vi "PID Online Autotuning (Step Open Loop).vi"(0 "setpoint":dbl(slide)=30.8641975308642 scale=0.0..100.0 scale format="%.1f", 1 "manipulated variable":dbl(slide)=30.8641975308642 scale=0.0..100.0 scale format="%.1f", 3 "autotuning parameters":T2={"type of controller"=0, "relay cycles"=3, "relay amplitude"=1.0, "control specifications"=2, "PV noise level"=0.1} {"PV noise level" format="%.2f"; "control specifications" items=["normal", "fast", "slow"]; "relay amplitude" format="%.2f"; "type of controller" items=["P", "PI", "PID"]}, 5 "process variable":dbl(slide)=19.583333333333336 scale=0.0..100.0 scale format="%.1f", 9 "PID gains in":T1={"proportional gain (Kc)"=1.0, "integral time (Ti, min)"=0.01, "derivative time (Td, min)"=0.0} {"derivative time (Td, min)" format="%.3f"; "integral time (Ti, min)" format="%.3f"; "proportional gain (Kc)" format="%.3f"}, 11 "dt (s)":dbl=-1.0 format="%.3f", 12 "reinitialize? (F)":bool, 13 "autotune? (F)":bool) -> (4 "setpoint out":dbl(slide)=30.8641975308642 scale=0.0..100.0 scale format="%.1f", 6 "process variable out":dbl(slide)=19.583333333333336 scale=0.0..100.0 scale format="%.1f", 8 "tuning completed?":bool, 10 "PID gains out":T1={"proportional gain (Kc)"=1.0, "integral time (Ti, min)"=0.01, "derivative time (Td, min)"=0.0} {"derivative time (Td, min)" format="%.3f"; "integral time (Ti, min)" format="%.3f"; "proportional gain (Kc)" format="%.3f"}, 14 "tuned PID gains":T1={"proportional gain (Kc)"=1.0, "integral time (Ti, min)"=0.01, "derivative time (Td, min)"=0.0} {"derivative time (Td, min)" format="%.3f"; "integral time (Ti, min)" format="%.3f"; "proportional gain (Kc)" format="%.3f"})   [LabVIEW 2017, in "NI_PID_autopid.lvlib"]
doc: "Controls the parameters of a PID controller based on the autotuning technique of the polymorphic instance you select. You can use this VI in applications with other PID VIs, such as PID or PID Advanced, to construct and tune a PID controller. You must manually select the polymorphic instance to use."
uses:
  <vilib>/addons/control/pid/NI_PID_autopid.lvlib
  <vilib>/addons/control/pid/autopid.llb/PID autotuning parameters.ctl
  <vilib>/addons/control/pid/autopid.llb/PID Autotuning Design (Auto).vi
  <vilib>/addons/control/pid/NI_PID_pid.lvlib
  <vilib>/ptbypt/NI_PtbyPt.lvlib
panel:
  # "Open Loop Step Response"
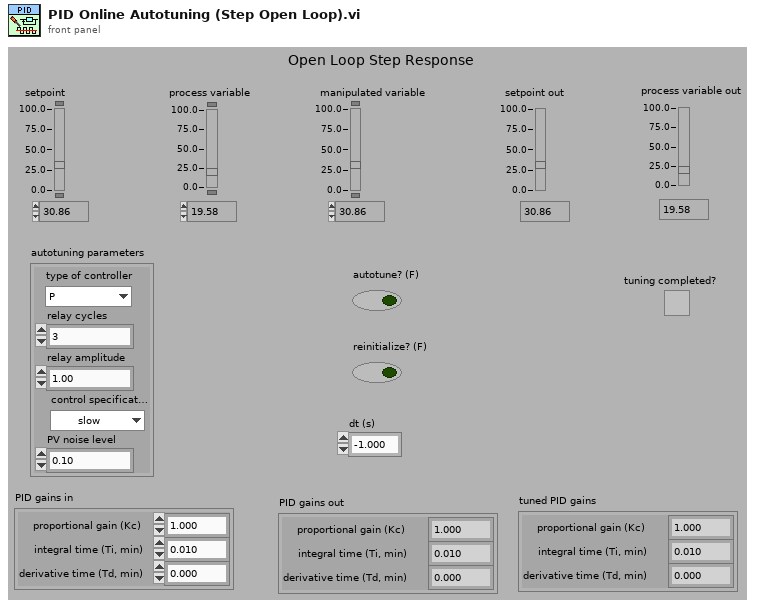
[diagram p1: front panel]
types:
  T1 = cluster{"proportional gain (Kc)":dbl, "integral time (Ti, min)":dbl, "derivative time (Td, min)":dbl}
  T2 = typedef "PID autotuning parameters.ctl" = cluster{"type of controller":u16, "relay cycles":i32, "relay amplitude":dbl, "control specifications":u16, "PV noise level":dbl}
  T3 = cluster{"Plant Gain (K)":dbl, "Time Constant (T)":dbl, "Dead Time (L)":dbl}
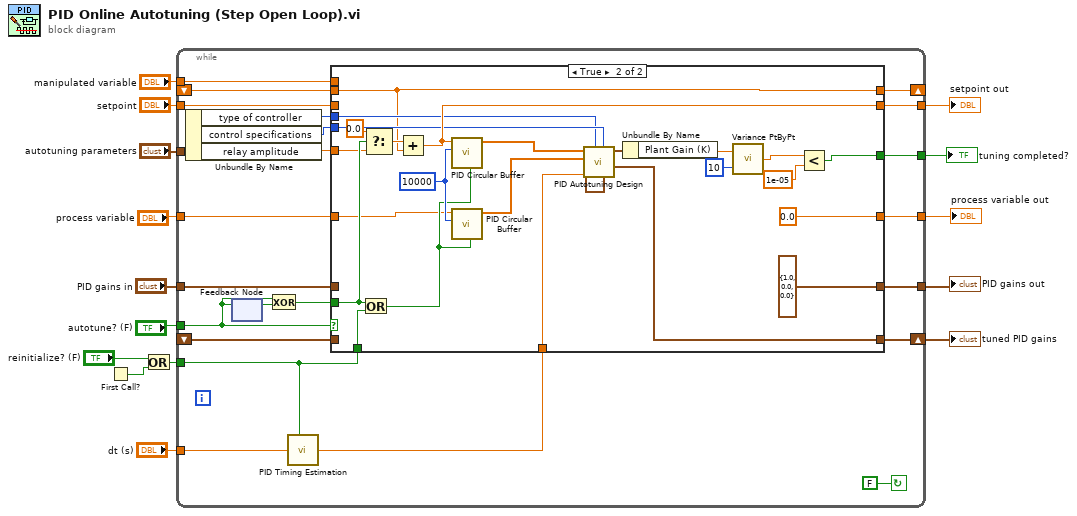
[diagram p0: block diagram]
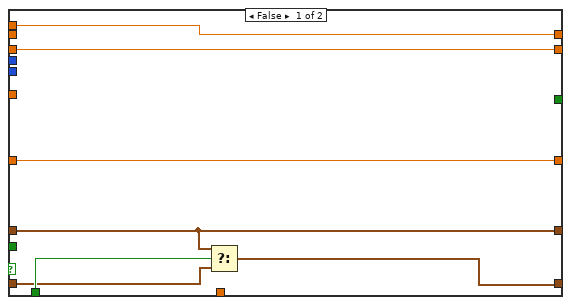
[diagram p2: hidden frame]
diagram:
  n1 = First Call?() -> (First Call?: T/F=w13:bool)
  n2 = Or(x="reinitialize? (F)", y=w13) -> (x .or. y?=w8:bool)
  n3 = while {
    tunnel: w8 -> [w18]
    tunnel: "dt (s)" -> [w19]
    tunnel: "process variable" -> [w34]
    tunnel: "autotuning parameters" -> [w36]
    tunnel: "PID gains in" -> [w29]
    tunnel: "setpoint" -> [w33]
    tunnel: "autotune? (F)" -> [w25]
    tunnel: "manipulated variable" -> [w35]
    tunnel: [w32] -> w5
    shift-right: [w31] -> _
    shift-left: _ -> [w30]
    tunnel: [w28] -> w4
    tunnel: [w27] -> w3
    shift-right: [w21] -> w2
    shift-left: _ -> [w20]
    tunnel: [w16] -> w1
    stop <- FALSE continue-if-true
    n4 = Unbundle By Name(w36) -> ("type of controller"=w23:u16, "control specifications"=w22:u16, "relay amplitude"=w37:dbl)
    n5 = feedback #1() -> (w26:bool)  [unwired: 1 in]
    n6 = feedback-in #1(w25) -> ()
    n7 = Exclusive Or(1:w26, 2:w25) -> (0:w24:bool)
    n8 = call <vilib>:"PID Timing Estimation.vi"("Initialize?"=w18, "dt (s) in"=w19) -> ("dt (s) out"=w17:dbl)  [unwired: 7 in]
    n9 = case shown="True" w25 {
      tunnel: w37 -> [_ w54]
      tunnel: w35 -> [w44 _]
      tunnel: w17 -> [_ w58]
      tunnel: w34 -> [w43 w61]
      tunnel: w18 -> [w42 w66]
      tunnel: [w45 w62] -> w32
      tunnel: w33 -> [w45 _]
      tunnel: [w44 w53] -> w31
      tunnel: w30 -> [_ w53]
      tunnel: [w39 T1 {"proportional gain (Kc)"=1.0, "integral time (Ti, min)"=0.0, "derivative time (Td, min)"=0.0} ("PID gains in")] -> w28
      tunnel: w29 -> [w39 _]
      tunnel: [w43 0.0 ("Process Variable")] -> w27
      tunnel: w24 -> [_ w63]
      tunnel: w23 -> [_ w56]
      tunnel: w22 -> [_ w57]
      tunnel: [w41 w55] -> w21
      tunnel: w20 -> [w40 _]
      tunnel: [_ w46] -> w16
      frame False {
        n10 = Select(t=w39, s=w42, f=w40) -> (s? t:f=w41:T1)
      }
      frame True {
        w67 = 10000 ("sample length")
        n11 = Or(x=w63, y=w66) -> (x .or. y?=w64:bool)
        n12 = Select(t=0.0, s=w63, f=w54) -> (s? t:f=w68:dbl)
        n13 = Add(x=w68, y=w53) -> (x+y=w62:dbl)
        n14 = call <vilib>:"PID Circular Buffer.vi"("initialize"=w64, "sample length"=w67, "input data point"=w62) -> ("Current Queue"=w60:dbl[])  [unwired: 7 in, 1 out]
        n15 = call <vilib>:"PID Circular Buffer.vi"("initialize"=w64, "sample length"=w67, "input data point"=w61) -> ("Current Queue"=w59:dbl[])  [unwired: 7 in, 1 out]
        n16 = call-poly <vilib>:"PID Autotuning Design.vi"("Ziegler-Nichols Speed"=w57, "Type of Controller"=w56, "dt (s)"=w58, "Response signal"=w59, "Stimulus signal"=w60) -> ("PID gains"=w55:T1, "Plant Parameters"=w51:T3)  [unwired: 3 in, 2 out]
        n17 = Unbundle By Name(w51) -> ("Plant Gain (K)"=w50:dbl)
        n18 = call <vilib>:"Variance PtByPt.vi"("x"=w50, "sample length"=10) -> ("variance"=w48:dbl)  [unwired: 1 in, 2 out]
        n19 = Less?(x=w48, y=1e-05) -> (x < y?=w46:bool)
      }
    }
  }
  "PID gains out" <- w4
  "process variable out" <- w3
  "setpoint out" <- w5
  "tuning completed?" <- w1
  "tuned PID gains" <- w2
